vi "Name.vi"(8 "error in (no error)":errorcluster, 10 "String in":string) -> (0 "error out":errorcluster, 1 "JSON name":string, 2 "Rest of string":string)   [LabVIEW 2011, in "JSON Value.lvclass"]
doc: "Splits a JSON value string into a name and it's value. Unescapes the name.\n\nCopyright 2012 James David Powell, Shaun Rumbell and Ton Plomp\nMore information on http://lavag.org/topic/16217-cr-json-labview"
uses:
  JSON Value.lvclass
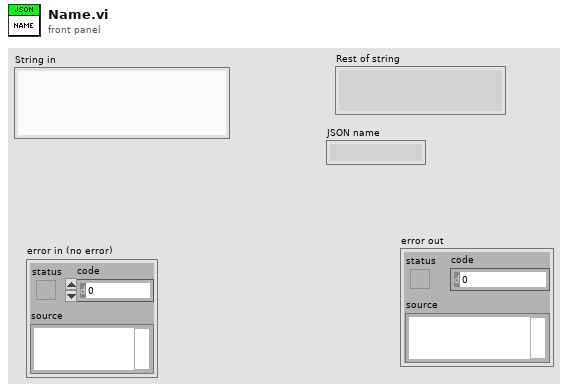
[diagram p1: front panel]
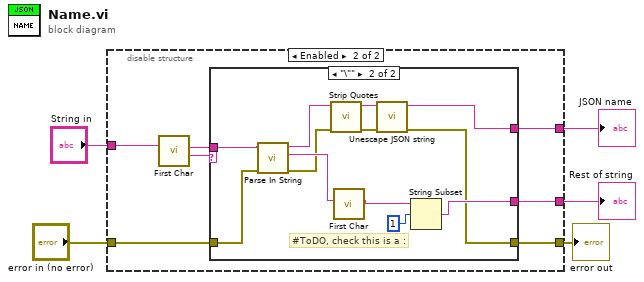
[diagram p0: block diagram]
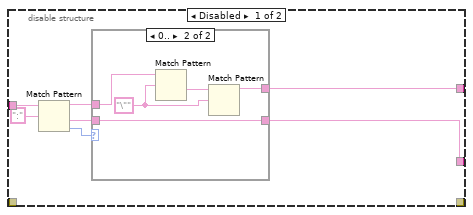
[diagram p2: hidden frame]
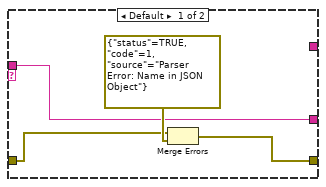
[diagram p4: hidden frame]
diagram:
  n1 = disable-structure shown="Enabled" {
    disable-tunnel: "String in" -> [w11 w25]
    disable-tunnel: [w9 w22] -> w4
    disable-tunnel: [w7 w21] -> w3
    disable-tunnel: [_ w20] -> w2
    disable-tunnel: "error in (no error)" -> [_ w19]
    frame Disabled {
      n2 = Match Pattern(string=w11, regular expression=":") -> (before substring=w10:string, after substring=w6:string, offset past match=w8:i32)  [unwired: 1 in, 1 out]
      n3 = case shown="0.." w8 {
        tunnel: w10 -> [w13 w18]
        tunnel: [_ w15] -> w9
        tunnel: [w13 w14] -> w7
        tunnel: w6 -> [_ w14]
        frame ..-1 {
          # "Pass through full string if\n\":\" not found (needed\nfor {} case.  -- JDP"
        }
        frame 0.. {
          w16 = "\"" ("regular expression")
          n4 = Match Pattern(string=w18, regular expression=w16) -> (after substring=w17:string)  [unwired: 1 in, 3 out]
          n5 = Match Pattern(string=w17, regular expression=w16) -> (before substring=w15:string)  [unwired: 1 in, 3 out]
        }
      }
    }
    frame Enabled {
      n6 = call "First Char.vi"("String in"=w25) -> ("First Char"=w24:string, "String"=w23:string)  [unwired: 9 in]
      n7 = case shown="\"\\\"\"" w24 {
        tunnel: w23 -> [w26 w41]
        tunnel: [_ w33] -> w22
        tunnel: [w26 w36] -> w21
        tunnel: [w27 w30] -> w20
        tunnel: w19 -> [w28 w40]
        frame Default {
          n8 = Merge Errors(w28, errorcluster {"status"=TRUE, "code"=1, "source"="Parser Error: Name in JSON Object"} ("error in")) -> (w27:errorcluster)
        }
        frame "\"" {
          # "#ToDO, check this is a :"
          n9 = call "Parse In String.vi"("error in (no error)"=w40, "Partial JSON (starting with quote)"=w41) -> ("error out"=w32:errorcluster, "Rest of JSON"=w39:string, "String (incl quotes)"=w35:string)  [unwired: 7 in]
          n10 = call "Strip Quotes.vi"("error in (no error)"=w32, "String"=w35) -> ("error out"=w31:errorcluster, "result string"=w34:string)  [unwired: 8 in]
          n11 = call "First Char.vi"("String in"=w39) -> ("String"=w37:string)  [unwired: 9 in, 1 out]
          n12 = call "Unescape JSON string.vi"("error in (no error)"=w31, "Text (with JSON escapes)"=w34) -> ("error out"=w30:errorcluster, "Text (unescaped)"=w33:string)  [unwired: 8 in]
          n13 = String Subset(string=w37, offset (0)=1 ("length (rest)")) -> (substring=w36:string)  [unwired: 1 in]
        }
      }
    }
  }
  "Rest of string" <- w3
  "JSON name" <- w4
  "error out" <- w2
